vi "Parse DateTime.vi"(11 "Line containing datetime":string="Date:15/04/21Tlmc:16:59:22") -> (1 "Success?":bool, 3 "time stamp":timestamp, 5 "Partial Date (use if error)":timestamp)   [LabVIEW 2018, in "Receipt Parsing.lvlib"]
uses:
  Receipt Parsing.lvlib
  <vilib>/Utility/miscctls.llb/LVDateTimeRec.ctl
  <vilib>/regexp/Match Regular Expression.xnode
panel:
  out "output cluster [debug]":T1
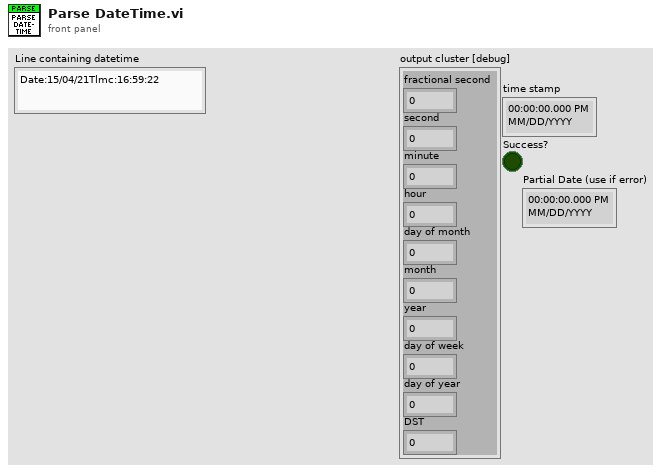
[diagram p1: front panel]
types:
  T1 = typedef "LVDateTimeRec.ctl" = cluster{"fractional second":dbl, "second":i32, "minute":i32, "hour":i32, "day of month":i32, "month":i32, "year":i32, "day of week":i32, "day of year":i32, "DST":i32}
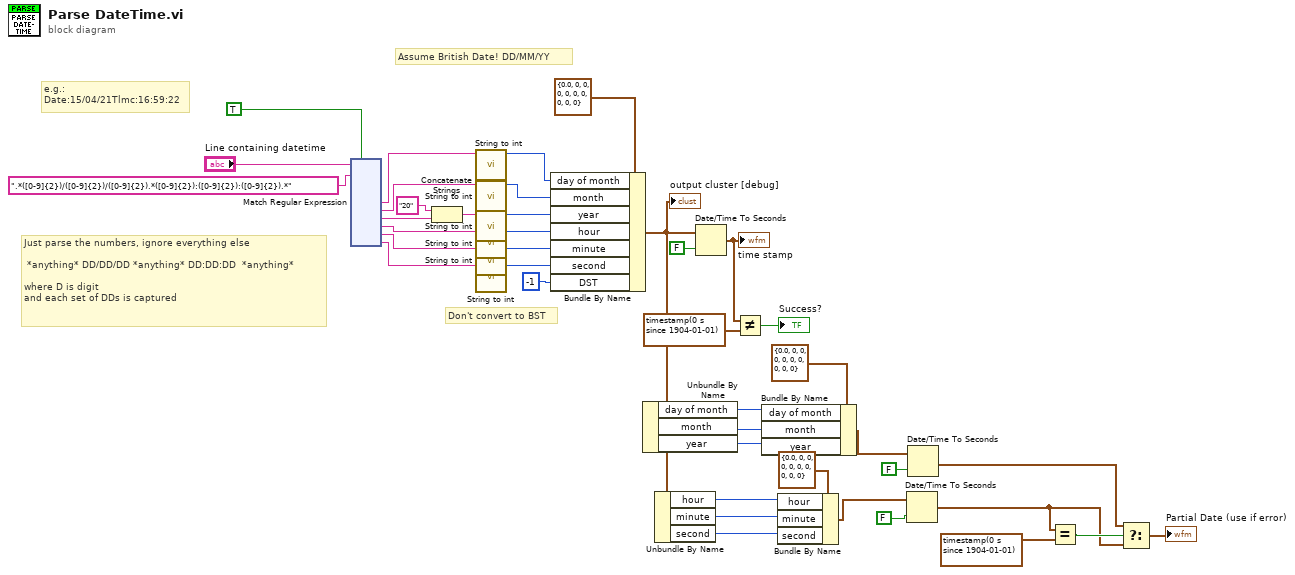
[diagram p0: block diagram]
diagram:
  # "Don't convert to BST"
  # "Just parse the numbers, ignore everything else\n\n *anything* DD/DD/DD *anything* DD:DD:DD  *anything*\n\nwhere D is digit\nand each set of DDs is captured"
  # "e.g.:\nDate:15/04/21Tlmc:16:59:22"
  # "Assume British Date! DD/MM/YY"
  n1 = xnode "Match Regular Expression"("input string"="Line containing datetime", "regular expression"=".*([0-9]{2})/([0-9]{2})/([0-9]{2}).*([0-9]{2}):([0-9]{2}):([0-9]{2}).*", "ignore case? (F)"=TRUE) -> ("submatch 1"=w37:string, "submatch 2"=w30:string, "submatch 3"=w25:string, "submatch 4"=w29:string, "submatch 5"=w28:string, "submatch 6"=w27:string)  [unwired: 3 in, 5 out]
  n2 = Concatenate Strings("20" ("string"), w25) -> (w23:string)
  n3 = call "String to int.vi"("Int as Text"=w37) -> ("Int"=w36:i32)  [unwired: 10 in]
  n4 = call "String to int.vi"("Int as Text"=w30) -> ("Int"=w31:i32)  [unwired: 10 in]
  n5 = call "String to int.vi"("Int as Text"=w23) -> ("Int"=w32:i32)  [unwired: 10 in]
  n6 = call "String to int.vi"("Int as Text"=w29) -> ("Int"=w33:i32)  [unwired: 10 in]
  n7 = call "String to int.vi"("Int as Text"=w28) -> ("Int"=w34:i32)  [unwired: 10 in]
  n8 = call "String to int.vi"("Int as Text"=w27) -> ("Int"=w35:i32)  [unwired: 10 in]
  n9 = Bundle By Name(cluster=T1 {"fractional second"=0.0, "second"=0, "minute"=0, "hour"=0, "day of month"=0, "month"=0, "year"=0, "day of week"=0, "day of year"=0, "DST"=0} ("date time rec"), "day of month"=w36, "month"=w31, "year"=w32, "hour"=w33, "minute"=w34, "second"=w35, "DST"=-1) -> (w15:T1)
  "output cluster [debug]" <- w15
  n10 = Unbundle By Name(w15) -> ("day of month"=w18:i32, "month"=w17:i32, "year"=w16:i32)
  n11 = Unbundle By Name(w15) -> ("hour"=w14:i32, "minute"=w13:i32, "second"=w12:i32)
  n12 = Date/Time To Seconds(1:FALSE ("is UTC (F)"), 2:w15) -> (0:w20:timestamp)
  "time stamp" <- w20
  n13 = Not Equal?(x=w20, y=timestamp(0 s since 1904-01-01) ("time stamp")) -> (x != y?=→"Success?":bool)
  n14 = Bundle By Name(cluster=T1 {"fractional second"=0.0, "second"=0, "minute"=0, "hour"=0, "day of month"=0, "month"=0, "year"=0, "day of week"=0, "day of year"=0, "DST"=0} ("date time rec"), "day of month"=w18, "month"=w17, "year"=w16) -> (w9:T1)
  n15 = Bundle By Name(cluster=T1 {"fractional second"=0.0, "second"=0, "minute"=0, "hour"=0, "day of month"=0, "month"=0, "year"=0, "day of week"=0, "day of year"=0, "DST"=0} ("date time rec"), "hour"=w14, "minute"=w13, "second"=w12) -> (w6:T1)
  n16 = Date/Time To Seconds(1:FALSE ("is UTC (F)"), 2:w6) -> (0:w2:timestamp)
  n17 = Date/Time To Seconds(1:FALSE ("is UTC (F)"), 2:w9) -> (0:w3:timestamp)
  n18 = Equal?(x=w2, y=timestamp(0 s since 1904-01-01) ("time stamp")) -> (x = y?=w4:bool)
  n19 = Select(t=w3, s=w4, f=w2) -> (s? t:f=→"Partial Date (use if error)":timestamp)
